vi "initialize.vi"(6 "timeout(-1)":i32, 7 "references":T1, 8 "error in (no error)":errorcluster, 11 "configuration":T3) -> (0 "error out":errorcluster)   [LabVIEW 2015, in "repub-dvr_nre.lvlib"]
doc: "Use this VI to set the running configuration and create any references needed by the application (or at the very least set the initialize flag to true). This VI as coded, will enqueue a command to the module main with the idea that references created there will remain in memory and not be garbage collected if the module is launched dynamically."
uses:
  repub-dvr_nre.lvlib
  private/_controls/input_command.ctl
  private/_controls/input.ctl
  _controls/error.ctl
  _controls/configuration.ctl
  private/_controls/output.ctl
  private/_controls/data.ctl
  _controls/references.ctl
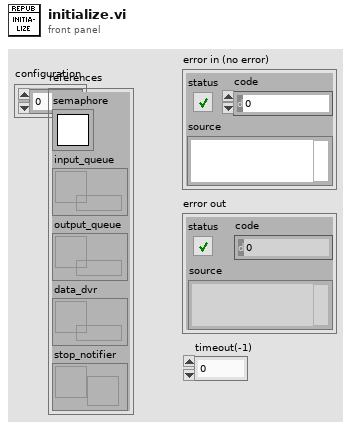
[diagram p1: front panel]
types:
  T1 = typedef "repub-dvr_nre.lvlib/references.ctl" = cluster{"semaphore":T2, "input_queue":refnum<queue>, "output_queue":refnum<queue>, "data_dvr":refnum<data-value>, "stop_notifier":refnum<notifier>}
  T2 = typedef "Semaphore RefNum" = refnum<k1>
  T3 = typedef "repub-dvr_nre.lvlib/configuration.ctl" = cluster{dbl}
  T4 = typedef "repub-dvr_nre.lvlib/error.ctl" = enum16{"<error>", "bad_command", "command_queue_timeout", "stop_notifier_timeout", "die_command_timeout", "<null>"}
  T5 = typedef "repub-dvr_nre.lvlib/input.ctl" = cluster{"command":T6, "data":variant}
  T6 = typedef "repub-dvr_nre.lvlib/input_command.ctl" = enum8{"<input_command>", "die", "initialize", "<null>"}
  T7 = typedef "repub-dvr_nre.lvlib/output.ctl" = cluster{"data":variant, "error":errorcluster}
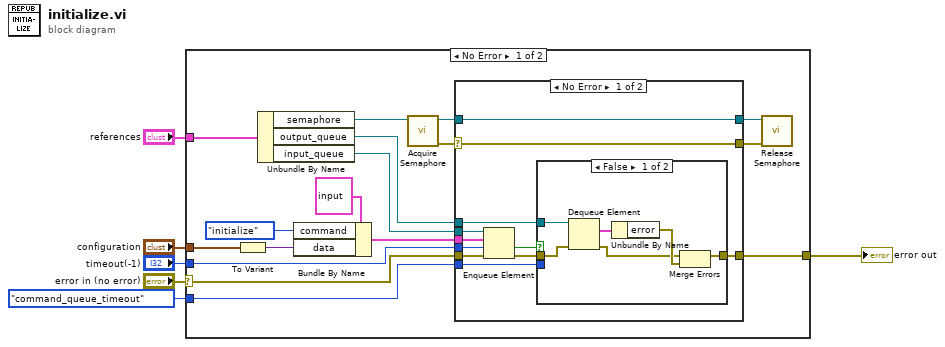
[diagram p0: block diagram]
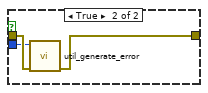
[diagram p2: hidden frame]
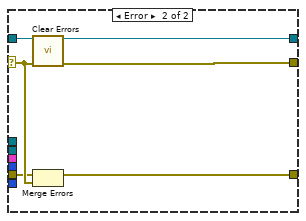
[diagram p3: hidden frame]
diagram:
  n1 = case shown="No Error" "error in (no error)" {
    selector: "error in (no error)" -> [w9 w49]
    tunnel: [w14 w49] -> w5
    tunnel: "timeout(-1)" -> [w20 _]
    tunnel: "configuration" -> [w13 _]
    tunnel: "references" -> [w11 _]
    tunnel: error."command_queue_timeout" ("error") -> [w7 _]
    frame No Error {
      n2 = To Variant(anything=w13) -> (Variant=w8:variant)
      n3 = Unbundle By Name(w11) -> ("semaphore"=w10:T2, "output_queue"=w21:refnum<queue>, "input_queue"=w23:refnum<queue>)
      n4 = Bundle By Name(cluster=T5 {"command"=enum."<input_command>", "data"=variant(cluster{"data":variant} {"data"=variant})} ("input"), "command"=input_command."initialize", "data"=w8) -> (w19:T5)
      n5 = call <vilib>:"Acquire Semaphore.vi"("semaphore"=w10) -> ("error out"=w22:errorcluster, "semaphore out"=w17:T2)  [unwired: 4 in, 1 out]
      n6 = case shown="No Error" w22 {
        selector: w22 -> [w27 w46]
        tunnel: w9 -> [w34 w45]
        tunnel: w23 -> [w33 _]
        tunnel: w21 -> [w31 _]
        tunnel: w20 -> [w30 _]
        tunnel: w19 -> [w29 _]
        tunnel: w17 -> [w28 w48]
        tunnel: [w28 w48] -> w16
        tunnel: [w27 w47] -> w15
        tunnel: [w25 w44] -> w14
        tunnel: w7 -> [w24 _]
        frame No Error {
          n7 = Enqueue Element(queue=w33, element=w29, timeout in ms (-1)=w30, error in (no error)=w34) -> (timed out?=w26:bool, error out=w32:errorcluster)  [unwired: 1 out]
          n8 = case shown="False" w26 {
            tunnel: w32 -> [w40 w43]
            tunnel: w31 -> [w39 _]
            tunnel: [w35 w42] -> w25
            tunnel: w24 -> [_ w41]
            frame False {
              n9 = Dequeue Element(queue=w39, error in (no error)=w40) -> (element=w38:T7, error out=w36:errorcluster)  [unwired: 1 in, 2 out]
              n10 = Unbundle By Name(w38) -> ("error"=w37:errorcluster)
              n11 = Merge Errors(w36, w37) -> (w35:errorcluster)
            }
            frame True {
              n12 = call "util_generate_error.vi"("error in (no error)"=w43, "error"=w41) -> ("error out"=w42:errorcluster)  [unwired: 9 in]
            }
          }
        }
        frame Error {
          n13 = call <vilib>:"Clear Errors.vi"("error in (no error)"=w46) -> ("error out"=w47:errorcluster)  [unwired: 5 in, 1 out]
          n14 = Merge Errors(w45, w46) -> (w44:errorcluster)
        }
      }
      n15 = call <vilib>:"Release Semaphore.vi"("error in (no error)"=w15, "semaphore"=w16) -> ()  [unwired: 4 in, 2 out]
    }
    frame Error {
    }
  }
  "error out" <- w5
